vi "Init.vi"(8 "error in (no error)":errorcluster, 10 "index":i32, 11 "BC_Steady_2D":refnum<class "NI_BC_Steady_2D.lvclass">) -> (0 "error out":errorcluster, 3 "initialized BC_Steady_2D":refnum<class "NI_BC_Steady_2D.lvclass">)   [LabVIEW 2017, in "NI_PDE.lvlib" / "NI_BC_Steady_2D.lvclass"]
uses:
  <vilib>/gmath/pde.llb/BCClass/BC_Steady_2D/NI_BC_Steady_2D.lvclass
  <vilib>/gmath/pde.llb/BCClass/Class Type.ctl
  <vilib>/gmath/pde.llb/BCClass/NI_BC.lvclass
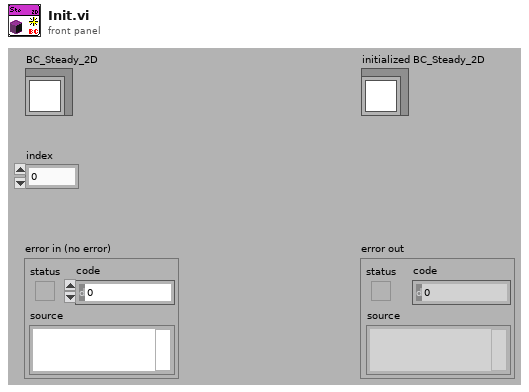
[diagram p1: front panel]
types:
  T1 = typedef "NI_PDE.lvlib/NI_BC.lvclass/Class Type.ctl" = i32
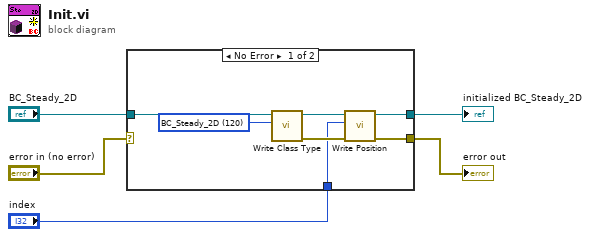
[diagram p0: block diagram]
diagram:
  n1 = case shown="No Error" "error in (no error)" {
    selector: "error in (no error)" -> [_ w14]
    tunnel: "BC_Steady_2D" -> [w12 w13]
    tunnel: [w8 w14] -> w4
    tunnel: [w9 w13] -> w3
    tunnel: "index" -> [w6 _]
    frame No Error {
      w11 = T1 120 items=["BC"=0, "BC_Steady"=100, "BC_Steady_2D"=120, "BC_Steady_2D_Numeric"=121, "BC_Steady_2D_VIRef"=122, "BC_Evolut"=200, "BC_Evolut_1D"=210, "BC_Evolut_1D_Numeric"=211, "BC_Evolut_1D_VIRef"=212, "BC_Evolut_2D"=220, "BC_Evolut_2D_Numeric"=221, "BC_Evolut_2D_VIRef"=222] ("BC class type")
      n2 = call-dynamic "Write Class Type.vi"("BC class type"=w11, "BC.lvclass in"=w12) -> ("error out"=w7:errorcluster, "BC.lvclass out"=w10:refnum<class "NI_BC_Steady_2D.lvclass">)  [unwired: 1 in, 7 out]
      n3 = call-dynamic "Write Position.vi"("error in (no error)"=w7, "BC position 2D"=w6, "BC_Steady_2D.lvclass in"=w10) -> ("error out"=w8:errorcluster, "BC_Steady_2D.lvclass out"=w9:refnum<class "NI_BC_Steady_2D.lvclass">)  [unwired: 7 out]
    }
    frame Error {
    }
  }
  "initialized BC_Steady_2D" <- w3
  "error out" <- w4
